vi "Get sensor serial number.vi"(1 "Geometry":string, 2 "Toplayer ID":string) -> (0 "Toplayer ID out":string)   [LabVIEW 2021, in "Stack.lvclass"]
uses:
  Stack.lvclass
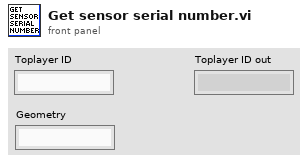
[diagram p1: front panel]
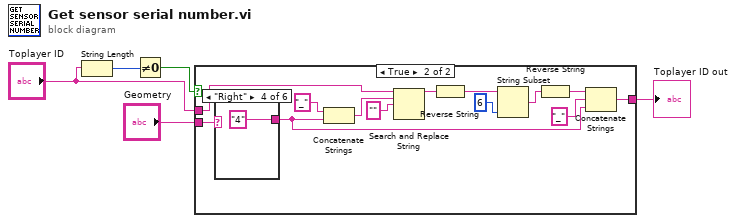
[diagram p0: block diagram]
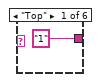
[diagram p3: hidden frame]
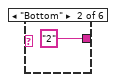
[diagram p4: hidden frame]
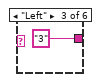
[diagram p5: hidden frame]
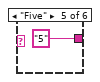
[diagram p6: hidden frame]
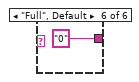
[diagram p7: hidden frame]
diagram:
  n1 = String Length(string="Toplayer ID") -> (length=w5:i32)
  n2 = Not Equal To 0?(x=w5) -> (x != 0?=w4:bool)
  n3 = case shown="True" w4 {
    tunnel: "Geometry" -> [_ w19]
    tunnel: [w6 w17] -> w3
    tunnel: "Toplayer ID" -> [w6 w12]
    frame False {
    }
    frame True {
      n4 = case shown="\"Right\"" w19 {
        tunnel: ["1" "2" "3" "4" "5" "0"] -> w11
        frame "Top" {
        }
        frame "Bottom" {
        }
        frame "Left" {
        }
        frame "Right" {
        }
        frame "Five" {
        }
        frame "Full", Default {
        }
      }
      n5 = Concatenate Strings("_" ("string"), w11) -> (w9:string)
      n6 = Search and Replace String(input string=w12, search string=w9, replace string="" ("replace string (\"\")")) -> (result string=w7:string)  [unwired: 5 in, 3 out]
      n7 = Reverse String(1:w7) -> (0:w16:string)
      n8 = String Subset(string=w16, length (rest)=6 ("length (rest)")) -> (substring=w14:string)  [unwired: 1 in]
      n9 = Reverse String(1:w14) -> (0:w13:string)
      n10 = Concatenate Strings(w13, "_" ("string"), w11) -> (w17:string)
    }
  }
  "Toplayer ID out" <- w3
